vi "solar_qtimer Set (Start).vi"(8 "error in (no error)":errorcluster, 10 "Start (F = Stop)":bool, 11 "QTimer Name":string) -> (0 "error out":errorcluster)   [LabVIEW 2018]
doc: "[DEPRECIATED] This sets the start/stop of the QTimer by name."
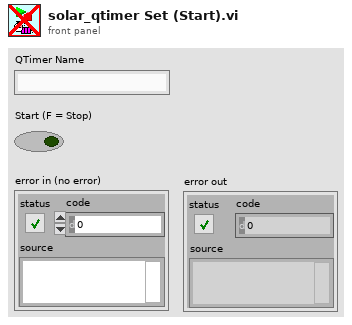
[diagram p1: front panel]
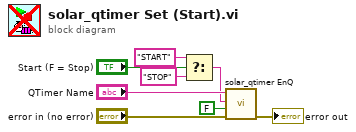
[diagram p0: block diagram]
diagram:
  n1 = Select(t="START" ("CMD (\"\")"), s="Start (F = Stop)", f="STOP" ("CMD (\"\")")) -> (s? t:f=w2:string)
  n2 = call "solar_qtimer EnQ.vi"("error in (no error)"="error in (no error)", "Create if not found? (F)"=FALSE, "CMD (\"\")"=w2, "QTimer Name"="QTimer Name") -> ("error out"=→"error out":errorcluster)  [unwired: 5 in, 2 out]
